vi "getAll.vi"(8 "error in (no error)":errorcluster, 11 "VISA Session":string) -> (0 "error out":errorcluster, 2 "SR7270 getAll":T1, 3 "VISA resource name out":refnum<visa-resource-name>)   [LabVIEW 2016, in "Instrument.SR7270.lvclass"]
uses:
  Instrument.SR7270.lvclass
  Typedefs/getAll.ctl
  Driver/SR7270 Drivers.lvlib
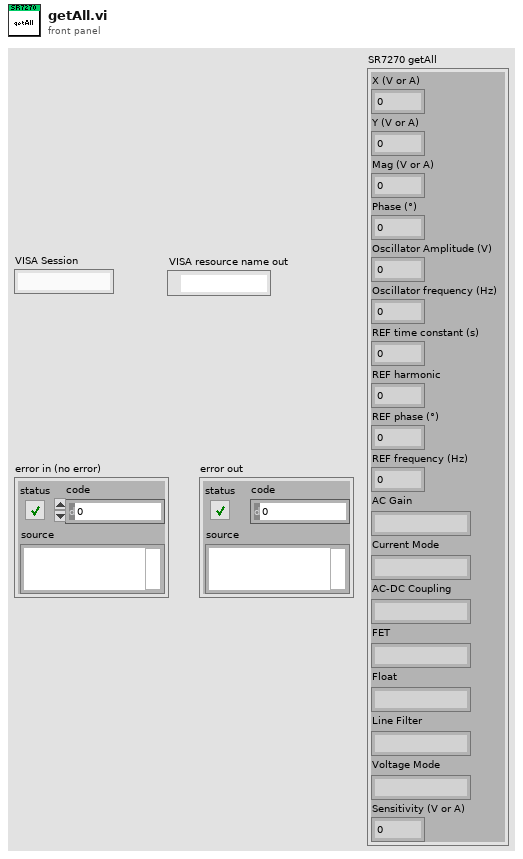
[diagram p1: front panel]
types:
  T1 = typedef "Instrument.SR7270.lvclass/getAll.ctl" = cluster{"X (V or A)":dbl, "Y (V or A)":dbl, "Mag (V or A)":dbl, "Phase (°)":dbl, "Oscillator Amplitude (V)":dbl, "Oscillator frequency (Hz)":dbl, "REF time constant (s)":dbl, "REF harmonic":u16, "REF phase (°)":dbl, "REF frequency (Hz)":dbl, "AC Gain":string, "Current Mode":string, "AC-DC Coupling":string, "FET":string, "Float":string, "Line Filter":string, "Voltage Mode":string, "Sensitivity (V or A)":dbl}
  T2 = typedef "SR7270 Drivers.lvlib/ACGAIN--enum.ctl" = enum16{"0 dB", "6 dB", "12 dB", "18 dB", "24 dB", "30 dB", "36 dB", "42 dB", "48 dB", "54 dB", "60 dB", "66 dB", "72 dB", "78 dB", "84 dB", "90 dB"}
  T3 = typedef "SR7270 Drivers.lvlib/IMODE--enum.ctl" = enum16{"Current Mode Off", "High bandwidth current mode", "Low noise current mode"}
  T4 = typedef "SR7270 Drivers.lvlib/DCCOUPLE--enum.ctl" = enum16{"AC coupled", "DC coupled"}
  T5 = typedef "SR7270 Drivers.lvlib/FET--enum.ctl" = enum16{"Bipolar", "FET"}
  T6 = typedef "SR7270 Drivers.lvlib/FLOAT--enum.ctl" = enum16{"Ground", "Float"}
  T7 = typedef "SR7270 Drivers.lvlib/LF--enum.ctl" = enum16{"Off", "60 Hz", "120 Hz", "60 & 120 Hz"}
  T8 = typedef "SR7270 Drivers.lvlib/VMODE--enum.ctl" = enum16{"Both Grounded", "A input only", "-B input only", "A-B differential"}
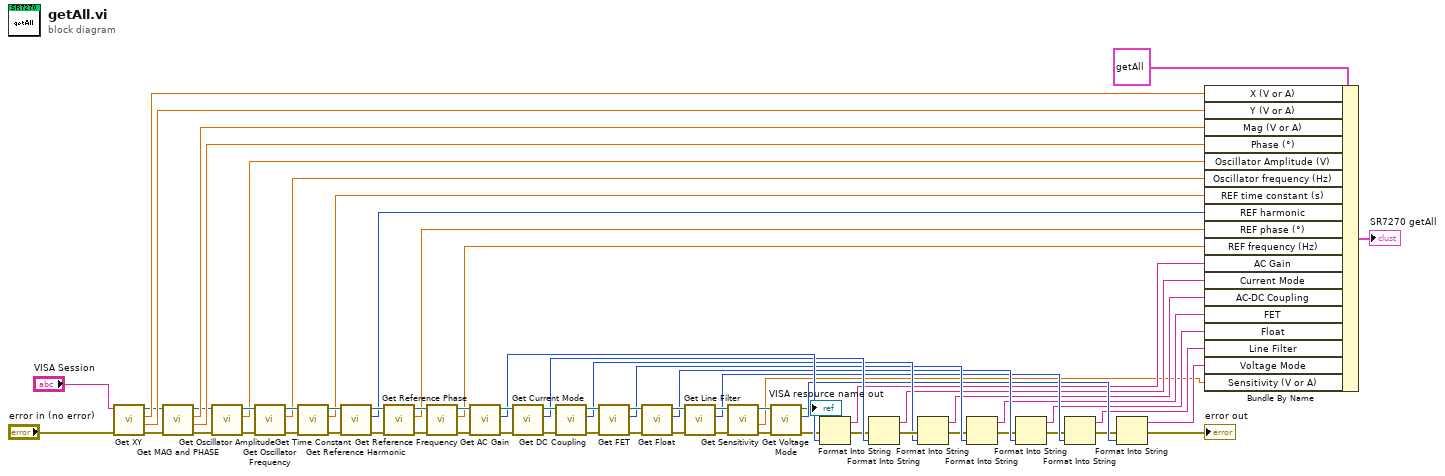
[diagram p0: block diagram]
diagram:
  n1 = call "Get XY.vi"("error in (no error)"="error in (no error)", "VISA resource name"="VISA Session") -> ("error out"=w62:errorcluster, "Y (V or A)"=w66:dbl, "X (V or A)"=w65:dbl, "VISA resource name out"=w63:refnum<visa-resource-name>)  [unwired: 6 in]
  n2 = call "Get MAG and PHASE.vi"("error in (no error)"=w62, "VISA resource name"=w63) -> ("error out"=w40:errorcluster, "Phase (°)"=w68:dbl, "Magnitude (V or A)"=w67:dbl, "VISA resource name out"=w39:refnum<visa-resource-name>)  [unwired: 6 in]
  n3 = call "Get Oscillator Amplitude.vi"("error in (no error)"=w40, "VISA resource name"=w39) -> ("error out"=w58:errorcluster, "Oscillator Amplitude (V)"=w27:dbl, "VISA resource name out"=w59:refnum<visa-resource-name>)  [unwired: 7 in]
  n4 = call "Get Oscillator Frequency.vi"("error in (no error)"=w58, "VISA resource name"=w59) -> ("error out"=w56:errorcluster, "Oscillator Frequency (Hz)"=w26:dbl, "VISA resource name out"=w57:refnum<visa-resource-name>)  [unwired: 7 in]
  n5 = call "Get Time Constant.vi"("error in (no error)"=w56, "VISA resource name"=w57) -> ("error out"=w54:errorcluster, "Time Constant (s)"=w25:dbl, "VISA resource name out"=w55:refnum<visa-resource-name>)  [unwired: 7 in]
  n6 = call "Get Reference Harmonic.vi"("error in (no error)"=w54, "VISA resource name"=w55) -> ("error out"=w52:errorcluster, "Harmonic"=w24:i32, "VISA resource name out"=w53:refnum<visa-resource-name>)  [unwired: 7 in]
  n7 = call "Get Reference Phase.vi"("error in (no error)"=w52, "VISA resource name"=w53) -> ("error out"=w50:errorcluster, "Phase (°)"=w23:dbl, "VISA resource name out"=w51:refnum<visa-resource-name>)  [unwired: 7 in]
  n8 = call "Get Reference Frequency.vi"("error in (no error)"=w50, "VISA resource name"=w51) -> ("error out"=w48:errorcluster, "Frequency (Hz)"=w22:dbl, "VISA resource name out"=w49:refnum<visa-resource-name>)  [unwired: 7 in]
  n9 = call "Get AC Gain.vi"("error in (no error)"=w48, "VISA resource name"=w49) -> ("error out"=w9:errorcluster, "AC Gain"=w38:T2, "VISA resource name out"=w47:refnum<visa-resource-name>)  [unwired: 7 in]
  n10 = call "Get Current Mode.vi"("error in (no error)"=w9, "VISA resource name"=w47) -> ("error out"=w8:errorcluster, "Current Mode"=w37:T3, "VISA resource name out"=w46:refnum<visa-resource-name>)  [unwired: 7 in]
  n11 = call "Get DC Coupling.vi"("error in (no error)"=w8, "VISA resource name"=w46) -> ("error out"=w7:errorcluster, "DC Coupling"=w35:T4, "VISA resource name out"=w45:refnum<visa-resource-name>)  [unwired: 7 in]
  n12 = call "Get FET.vi"("error in (no error)"=w7, "VISA resource name"=w45) -> ("error out"=w6:errorcluster, "FET Mode"=w34:T5, "VISA resource name out"=w44:refnum<visa-resource-name>)  [unwired: 7 in]
  n13 = call "Get Float.vi"("error in (no error)"=w6, "VISA resource name"=w44) -> ("error out"=w5:errorcluster, "Float Mode"=w31:T6, "VISA resource name out"=w43:refnum<visa-resource-name>)  [unwired: 7 in]
  n14 = call "Get Line Filter.vi"("error in (no error)"=w5, "VISA resource name"=w43) -> ("error out"=w4:errorcluster, "Line Frequency Rejection"=w30:T7, "VISA resource name out"=w42:refnum<visa-resource-name>)  [unwired: 7 in]
  n15 = call "Get Sensitivity.vi"("error in (no error)"=w4, "VISA resource name"=w42) -> ("error out"=w3:errorcluster, "Sensitivity (A or V)"=w14:dbl, "VISA resource name out"=w41:refnum<visa-resource-name>)  [unwired: 6 in, 1 out]
  n16 = call "Get Voltage Mode.vi"("error in (no error)"=w3, "VISA resource name"=w41) -> ("error out"=w2:errorcluster, "Voltage Mode"=w29:T8, "VISA resource name out"=→"VISA resource name out":refnum<visa-resource-name>)  [unwired: 7 in]
  n17 = Format Into String(error in=w2, w38) -> (resulting string=w21:string, error out=w32:errorcluster)  [unwired: 2 in]
  n18 = Format Into String(error in=w32, w37) -> (resulting string=w20:string, error out=w36:errorcluster)  [unwired: 2 in]
  n19 = Format Into String(error in=w36, w35) -> (resulting string=w19:string, error out=w33:errorcluster)  [unwired: 2 in]
  n20 = Format Into String(error in=w33, w34) -> (resulting string=w18:string, error out=w13:errorcluster)  [unwired: 2 in]
  n21 = Format Into String(error in=w13, w31) -> (resulting string=w17:string, error out=w12:errorcluster)  [unwired: 2 in]
  n22 = Format Into String(error in=w12, w30) -> (resulting string=w16:string, error out=w11:errorcluster)  [unwired: 2 in]
  n23 = Format Into String(error in=w11, w29) -> (resulting string=w15:string, error out=→"error out":errorcluster)  [unwired: 2 in]
  n24 = Bundle By Name(cluster=T1 {"X (V or A)"=0.0, "Y (V or A)"=0.0, "Mag (V or A)"=0.0, "Phase (°)"=0.0, "Oscillator Amplitude (V)"=0.0, "Oscillator frequency (Hz)"=0.0, "REF time constant (s)"=0.0, "REF harmonic"=0, "REF phase (°)"=0.0, "REF frequency (Hz)"=0.0, "AC Gain"="", "Current Mode"="", "AC-DC Coupling"="", "FET"="", "Float"="", "Line Filter"="", "Voltage Mode"="", "Sensitivity (V or A)"=0.0}, "X (V or A)"=w65, "Y (V or A)"=w66, "Mag (V or A)"=w67, "Phase (°)"=w68, "Oscillator Amplitude (V)"=w27, "Oscillator frequency (Hz)"=w26, "REF time constant (s)"=w25, "REF harmonic"=w24, "REF phase (°)"=w23, "REF frequency (Hz)"=w22, "AC Gain"=w21, "Current Mode"=w20, "AC-DC Coupling"=w19, "FET"=w18, "Float"=w17, "Line Filter"=w16, "Voltage Mode"=w15, "Sensitivity (V or A)"=w14) -> (→"SR7270 getAll":T1)
